vi "2.1 Read Sensor Data.vi"() -> ()   [LabVIEW 2011]
uses:
  2 Typedefs/indicator LED.ctl
  2 Globals/2 Global.vi
panel:
  out "incoming sentence":string
  in  "stop":bool
  out "Current Status":enum16{"Waiting", "Reading", "Time Out!"}(ring)
  in  "VISA resource name":refnum<visa-resource-name>="COM1"
  in  "error in (no error)":errorcluster
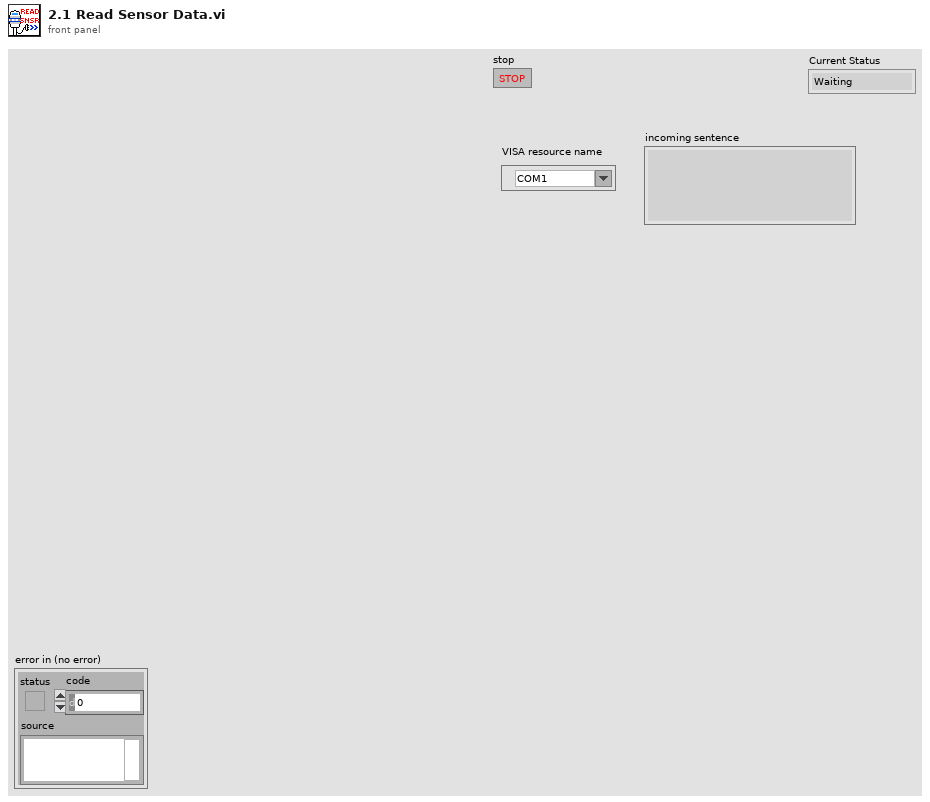
[diagram p1: front panel]
types:
  T1 = typedef "indicator LED.ctl" = bool
  T2 = typedef "generalized sensor status.ctl" = cluster{"Sensor Connected":T1, "Sensor Initialized":T1, "Sensor OK":T1, "Latest Error String":string}
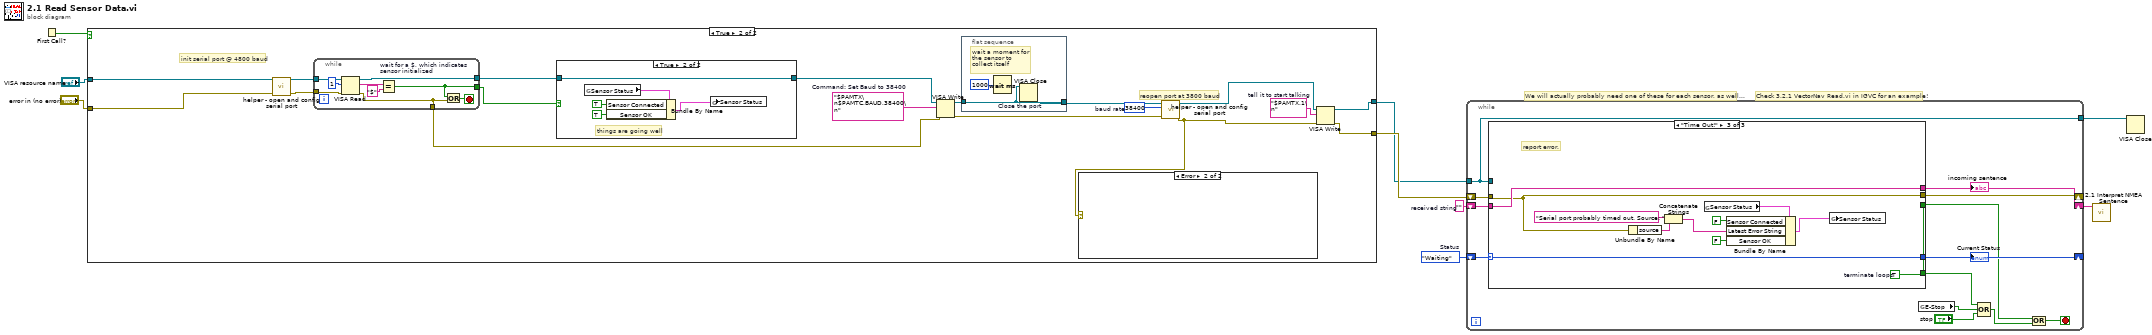
[diagram p0: block diagram]
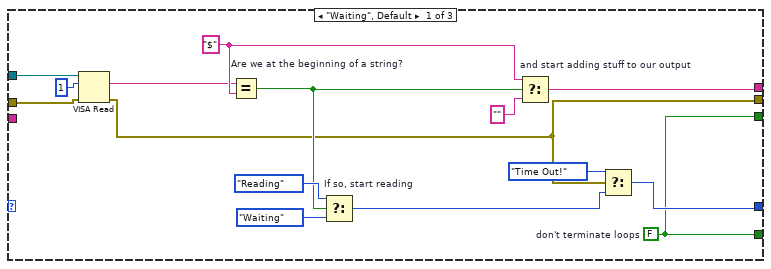
[diagram p2: hidden frame]
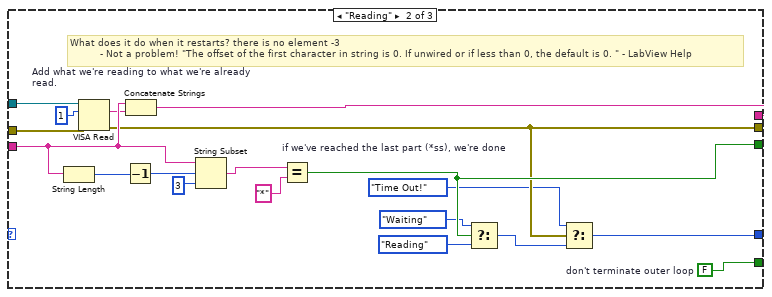
[diagram p3: hidden frame]
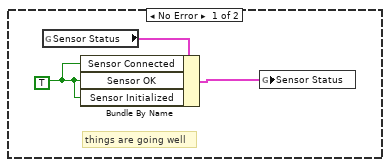
[diagram p5: hidden frame]
diagram:
  w1 = enum16{"Waiting", "Reading", "Time Out!"}."Waiting"  # Status
  w3 = ""  # received string
  # "Check 3.2.1 VectorNav Read.vi in IGVC for an example!"
  # "We will actually probably need one of these for each sensor, as well..."
  n1 = First Call?() -> (First Call?: T/F=w7:bool)
  n2 = case shown="True" w7 {
    tunnel: [w11 w18] -> w6
    tunnel: [w10 w12] -> w8
    tunnel: "VISA resource name" -> [w11 w17]
    tunnel: "error in (no error)" -> [w10 w16]
    frame False {
    }
    frame True {
      w19 = "$PAMTX,1\n"  # tell it to start talking
      w24 = u32 38400  # baud rate
      w28 = "$PAMTX\n$PAMTC,BAUD,38400\n"  # Command: Set Baud to 38400
      # "reopen port at 3800 baud"
      # "init serial port @ 4800 baud"
      n3 = call "helper - open and config serial port.vi"("error in (no error)"=w16, "VISA Refnum in"=w17) -> ("error out"=w15:errorcluster, "VISA Refnum out"=w21:refnum<visa-resource-name>)  [unwired: 8 in]
      n4 = while {
        tunnel: w21 -> [w40]
        tunnel: [w37] -> w29
        tunnel: [w39] -> w26
        tunnel: w15 -> [w38]
        tunnel: [w35] -> w14
        stop <- w36 stop-if-true
        n5 = VISA Read(VISA resource name=w40, byte count=u32 1, error in (no error)=w38) -> (VISA resource name out=w39:refnum<visa-resource-name>, read buffer=w42:string, error out=w35:errorcluster)  [unwired: 1 out]
        n6 = Equal? "wait for a $, which indicates\nsensor initialized"(x=w42, y="$" ("x")) -> (x = y?=w37:bool)
        n7 = Or(x=w37, y=w35) -> (x .or. y?=w36:bool)
      }
      n8 = case shown="True" w29 {
        tunnel: [w44 w45] -> w27
        tunnel: w26 -> [w44 w45]
        frame False {
        }
        frame True {
          # "things are going well"
          n9 = global read "2 Global.vi" "Sensor Status"() -> (w48:T2)
          n10 = Bundle By Name(cluster=w48, "Sensor Connected"=T1 TRUE, "Sensor OK"=T1 TRUE) -> (w49:T2)
          n11 = global write "2 Global.vi" "Sensor Status"(w49) -> ()
        }
      }
      n12 = VISA Write(VISA resource name=w27, write buffer=w28, error in (no error)=w14) -> (VISA resource name out=w25:refnum<visa-resource-name>, error out=w23:errorcluster)  [unwired: 1 out]
      n13 = flat-sequence {
        tunnel: [w33] -> w22
        tunnel: w25 -> [w33]
        frame #0 {
          # "wait a moment for\nthe sensor to \ncollect itself"
          n14 = Wait (ms)(milliseconds to wait=u32 1000) -> ()  [unwired: 1 out]
          n15 = VISA Close "Close the port"(VISA resource name=w33) -> ()  [unwired: 1 in, 1 out]
        }
      }
      n16 = call "helper - open and config serial port.vi"("error in (no error)"=w23, "baud rate"=w24, "VISA Refnum in"=w22) -> ("error out"=w13:errorcluster, "VISA Refnum out"=w20:refnum<visa-resource-name>)  [unwired: 7 in]
      n17 = case shown="Error" w13 {
        frame No Error {
          w30 = T1 TRUE ("Sensor OK")
          # "things are going well"
          n18 = global read "2 Global.vi" "Sensor Status"() -> (w31:T2)
          n19 = Bundle By Name(cluster=w31, "Sensor Connected"=w30, "Sensor OK"=w30, "Sensor Initialized"=w30) -> (w32:T2)
          n20 = global write "2 Global.vi" "Sensor Status"(w32) -> ()
        }
        frame Error {
        }
      }
      n21 = VISA Write(VISA resource name=w20, write buffer=w19, error in (no error)=w13) -> (VISA resource name out=w18:refnum<visa-resource-name>, error out=w12:errorcluster)  [unwired: 1 out]
    }
  }
  n22 = while {
    shift-right: [w50] -> w2
    shift-left: w3 -> [w62]
    shift-right: [w59] -> _
    shift-left: w1 -> [w61]
    tunnel: w6 -> [w57]
    tunnel: [w57] -> w9
    shift-right: [w55] -> _
    shift-left: w8 -> [w56]
    stop <- w60 stop-if-true
    n23 = case shown="\"Time Out!\"" w61 {
      selector: w61 -> [_ _ w107]
      tunnel: w62 -> [_ w90 w106]
      tunnel: [w73 w96 w106] -> w50
      tunnel: [w67 w81 w107] -> w59
      tunnel: [w63 w87 w97] -> w58
      tunnel: w57 -> [w70 w85 _]
      tunnel: w56 -> [w68 w83 w105]
      tunnel: [w65 w82 w105] -> w55
      tunnel: [w63 w78 w97] -> w51
      frame "Waiting", Default {
        w63 = FALSE  # don't terminate loops
        w72 = "$" ("x")
        n24 = VISA Read(VISA resource name=w70, byte count=u32 1, error in (no error)=w68) -> (read buffer=w71:string, error out=w65:errorcluster)  [unwired: 2 out]
        n25 = Equal? "Are we at the beginning of a string?"(x=w71, y=w72) -> (x = y?=w74:bool)
        n26 = Select "If so, start reading"(t=enum16{"Waiting", "Reading", "Time Out!"}."Reading", s=w74, f=enum16{"Waiting", "Reading", "Time Out!"}."Waiting" ("Current Status")) -> (s? t:f=w66:enum16{"Waiting", "Reading", "Time Out!"})
        n27 = Select "and start adding stuff to our output"(t=w72, s=w74, f="") -> (s? t:f=w73:string)
        n28 = Select(t=enum16{"Waiting", "Reading", "Time Out!"}."Time Out!", s=w65, f=w66) -> (s? t:f=w67:enum16{"Waiting", "Reading", "Time Out!"})
      }
      frame "Reading" {
        w78 = FALSE  # don't terminate outer loop
        # "What does it do when it restarts? there is no element -3\n          - Not a problem! \"The offset of the first character in string is 0. If unwired or if less than 0, the default is 0. \" - LabView Help"
        n29 = String Length(string=w90) -> (length=w95:i32)
        n30 = VISA Read(VISA resource name=w85, byte count=u32 1, error in (no error)=w83) -> (read buffer=w89:string, error out=w82:errorcluster)  [unwired: 2 out]
        n31 = Decrement(x=w95) -> (x-1=w94:i32)
        n32 = Concatenate Strings "Add what we're reading to what we're already read."(w90, w89) -> (w96:string)
        n33 = String Subset(string=w90, offset (0)=w94, length (rest)=3 ("length (rest)")) -> (substring=w92:string)
        n34 = Equal? "if we've reached the last part (*ss), we're done"(x=w92, y="*") -> (x = y?=w87:bool)
        n35 = Select(t=enum16{"Waiting", "Reading", "Time Out!"}."Waiting", s=w87, f=enum16{"Waiting", "Reading", "Time Out!"}."Reading" ("Status")) -> (s? t:f=w80:enum16{"Waiting", "Reading", "Time Out!"})
        n36 = Select(t=enum16{"Waiting", "Reading", "Time Out!"}."Time Out!", s=w82, f=w80) -> (s? t:f=w81:enum16{"Waiting", "Reading", "Time Out!"})
      }
      frame "Time Out!" {
        w97 = TRUE  # terminate loops
        # "report error."
        n37 = Unbundle By Name(w105) -> ("source"=w99:string)
        n38 = Concatenate Strings("Serial port probably timed out. Source: " ("string"), w99) -> (w100:string)
        n39 = global read "2 Global.vi" "Sensor Status"() -> (w103:T2)
        n40 = Bundle By Name(cluster=w103, "Sensor Connected"=T1 FALSE, "Latest Error String"=w100, "Sensor OK"=T1 FALSE) -> (w102:T2)
        n41 = global write "2 Global.vi" "Sensor Status"(w102) -> ()
      }
    }
    "Current Status" <- w59
    "incoming sentence" <- w50
    n42 = global read "2 Global.vi" "E-Stop"() -> (w53:bool)
    n43 = Compound Arithmetic op=OR(w51, w53, "stop") -> (w52:bool)
    n44 = Compound Arithmetic op=OR(w58, w52) -> (w60:bool)
  }
  n45 = call "2.1 Interpret NMEA Sentence.vi"("NMEA Sentence"=w2) -> ()  [unwired: 11 in]
  n46 = VISA Close(VISA resource name=w9) -> ()  [unwired: 1 in, 1 out]
